vi "Collect Vel APP_Ret and dt_us.vi"(0 "reference in":refnum<class "metadata.lvclass">, 5 "error in (no error)":errorcluster) -> (14 "reference out":refnum<class "metadata.lvclass">, 15 "Real dt (sec)":dbl, 16 "Vel_app (nm/s) out":dbl=3.0 min=3.0 max=5000000.0 step=1.0 format="%#.7f", 17 "Vel_ret (nm/s) out":dbl=3.0 min=3.0 max=5000000.0 step=1.0 format="%#.7f", 19 "error out":errorcluster)   [LabVIEW 2019, in "metadata.lvclass"]
uses:
  metadata.lvclass
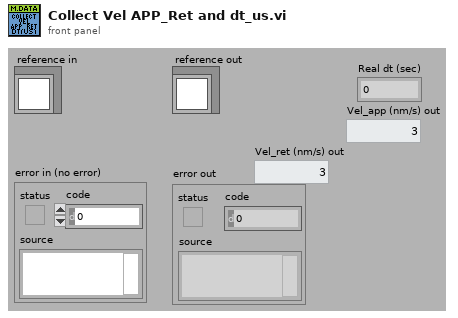
[diagram p1: front panel]
types:
  T1 = typedef "metadata.lvclass/ObjectAttributes.ctl" = cluster{"MyAttribute":dbl, "System Control":T2, "file info":T3, "Sample info":T4, "Cantilever info":T5, "XYZ piezos":T6, "Mapping":T7, "Fcurve segment":T8[], "Fast fpga segment":T10, "Chirp":T11, "precision (6)":i16, "width (-)":i16, "Metadata":T12, "config filepath":path, "Section names []":string[], "Property names []":string[], "nb elements":u16}
  T2 = typedef "metadata.lvclass/System control parameters.ctl" = cluster{"FPGA SW version":string, "TDMS file version":string, "Instrument":string, "Instrument model":string, "Instrument scanner":string, "Instrument clockrate (Mhz)":string, "Instrument tick time (us)":string}
  T3 = typedef "metadata.lvclass/File info parameters.ctl" = cluster{"Time Stamp":timestamp, "Filename":string, "Filepath":path, "User":string, "Experiment_name":string, "Curve_id":string, "number_segments":u8, "number_consecutive_scans":u32}
  T4 = typedef "metadata.lvclass/Sample info parameters.ctl" = cluster{"Sample name":string, "Sample species":string}
  T5 = typedef "metadata.lvclass/Cantilever info parameters.ctl" = cluster{"spring constant calib method":string, "invOLS calib method":string, "thermal calib deflection channel":string, "model":string, "shape":string, "tip geometry":string, "Laser sum (V)":dbl, "Laser power (mA)":dbl, "invOLS_(nm/V)":dbl, "spring constant nominal (N/m)":dbl, "spring constant calib (N/m)":dbl, "resosnance frequency air calib (Hz)":dbl, "resosnance frequency calib (Hz)":dbl, "quality factor":dbl, "Acoefficident_GCI_(nN.s^1.3/m)":dbl, "half angle (deg)":dbl, "tip radius (m)":dbl, "tip height (m)":dbl, "system mount angle (deg)":dbl}
  T6 = typedef "metadata.lvclass/XYZ piezos parameters.ctl" = cluster{"X stage piezo sensitivity (nm/V)":dbl, "X stage piezo gain":dbl, "X velocity (V/tick)":dbl, "X closed loop":bool, "Y stage piezo sensitivity (nm/V)":dbl, "Y stage piezo gain":dbl, "Y velocity (V/tick)":dbl, "Y closed loop":bool, "Z stage piezo sensitivity (nm/V)":dbl, "Z stage piezo gain":dbl, "Z closed loop":bool, "X position (V)":dbl, "Y position (V)":dbl}
  T7 = typedef "metadata.lvclass/Mapping parameters.ctl" = cluster{"Mapping":bool, "index":u16, "position row":u16, "position column":u16, "next position row":i16, "next position column":i16, "X initial position (V)":dbl, "Y initial position (V)":dbl, "X step size (V)":dbl, "Y step size (V)":dbl}
  T8 = typedef "metadata.lvclass/Fcurve segment.ctl" = cluster{"type":T9, "fast_fpga_trigger":bool, "nb":u8, "duration (ticks)":i64, "nb points":i32, "sampling rate (S/s)":u32, "Zpiezo control out":string, "initial deflection (V)":dbl, "relative setpoint":bool, "setpoint on":bool, "setpoint (V)":dbl, "setpoint trigger channel":string, "velocity (V/tick)":dbl, "Z position setpoint trigger (V)":dbl, "Z retract length (V)":dbl, "dec factor":u32}
  T9 = typedef "metadata.lvclass/Segment type--combobox.ctl" = string
  T10 = typedef "metadata.lvclass/fast fpga segment parameters.ctl" = cluster{"Fast start time trigger":timestamp, "nb_points":u32, "sampling_rate_(S/s)":u32, "duration_(ticks)":u32}
  T11 = typedef "metadata.lvclass/Chirp added parameters.ctl" = cluster{"f start (Hz)":dbl, "f end (Hz)":dbl, "Sweep type":string}
  T12 = typedef "metadata.lvclass/Metadata output --cluster.ctl" = cluster{"Property Names":string[], "Property Values":variant[]}
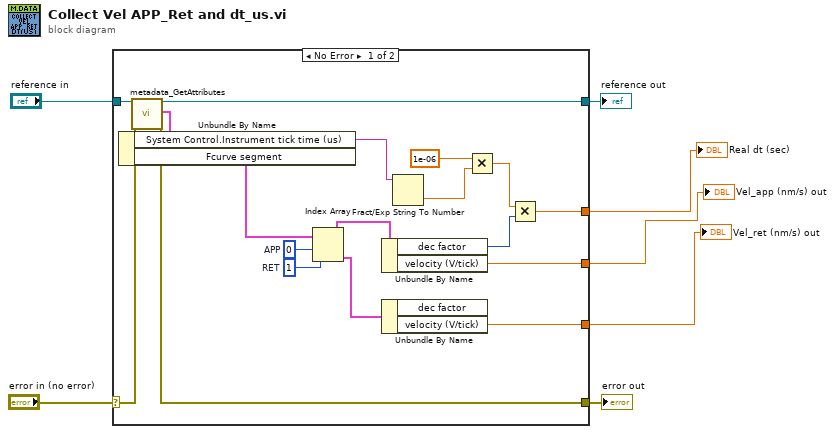
[diagram p0: block diagram]
diagram:
  n1 = case shown="No Error" "error in (no error)" {
    selector: "error in (no error)" -> [w25 w27]
    tunnel: [w24 w27] -> w6
    tunnel: [w23 w26] -> w4
    tunnel: "reference in" -> [w21 w26]
    tunnel: [w13 _] -> w3
    tunnel: [w9 _] -> w2
    tunnel: [w8 _] -> w1
    frame No Error {
      w11 = 1  # RET
      w12 = 0  # APP
      n2 = call "metadata_GetAttributes.vi"("reference in"=w21, "error in (no error)"=w25) -> ("reference out"=w23:refnum<class "metadata.lvclass">, "attributes"=w22:T1, "error out"=w24:errorcluster)  [unwired: 14 in, 1 out]
      n3 = Unbundle By Name(w22) -> ("System Control.Instrument tick time (us)"=w20:string, "Fcurve segment"=w17:T8[])
      n4 = Index Array(array=w17, index #1=w12, index #2=w11) -> (element #1=w16:T8, element #2=w10:T8)
      n5 = Unbundle By Name(w16) -> ("dec factor"=w15:u32, "velocity (V/tick)"=w8:dbl)
      n6 = Unbundle By Name(w10) -> ("velocity (V/tick)"=w9:dbl)  [unwired: 1 out]
      n7 = Fract/Exp String To Number(string=w20) -> (number=w19:dbl)  [unwired: 3 in, 1 out]
      n8 = Multiply(x=1e-06, y=w19) -> (x*y=w14:dbl)
      n9 = Multiply(x=w14, y=w15) -> (x*y=w13:dbl)
    }
    frame Error {
    }
  }
  "error out" <- w6
  "reference out" <- w4
  "Real dt (sec)" <- w3
  "Vel_app (nm/s) out" <- w1
  "Vel_ret (nm/s) out" <- w2
